vi "Ext.vi"(8 "error in (no error)":errorcluster, 9 "Val":variant, 10 "Tag":u16, 11 "Pulse in":refnum<class "Rigol DG822 Pulse.lvclass">) -> (0 "error out":errorcluster, 1 "Parsed":variant, 3 "Pulse out":refnum<class "Rigol DG822 Pulse.lvclass">)   [LabVIEW 2021, in "Rigol DG822 UI.lvlib" / "Rigol DG822 Pulse.lvlib" / "Rigol DG822 Pulse.lvclass"]
uses:
  Rigol DG822 Pulse.lvclass
  Rigol DG822 UI/lib/controls.llb/WaveformExtCall.ctl
  Rigol DG822 UI/lib/controls.llb/WaveformParamTags.ctl
  Rigol DG822 Pulse.lvclass/Rigol DG822 Pulse.ctl
  Rigol DG822 UI/lib/controls.llb/AllWaveformDataCluster.ctl
  Rigol DG822 UI/lib/controls.llb/DataCluster.ctl
  Rigol DG822 UI/lib/controls.llb/FT Controls Cluster.ctl
  Rigol DG822 UI/lib/controls.llb/String Indicators Cluster.ctl
  General/Files/lvlibp/Actors.lvlibp/Actors/Actors/Actors.lvclass
  D:/LabVIEW/General/Files/lvlibp/Actors.lvlibp/Actors/Actors/Actors.lvclass
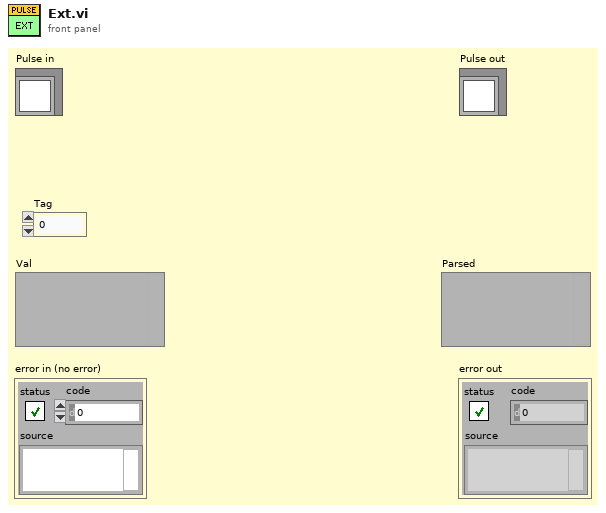
[diagram p1: front panel]
types:
  T1 = typedef "WaveformExtCall.ctl" = enum16{"Freq", "Period", "Ampl", "HighL", "Offset", "LowL", "Phase", "Duty", "Width", "RisEdge", "FallEdge", "Home", "InitData"}
  T2 = typedef "WaveformParamTags.ctl" = enum16{"Freq", "Period", "Ampl", "HighL", "Offset", "LowL", "Phase", "Duty", "Width", "RisEdge", "FallEdge"}
  T3 = cluster{"ParamTags":T2, "ParamTags 2":T2, "ParamTags 3":T2}
  T4 = typedef "AllWaveformDataCluster.ctl" = cluster{"Data":T5, "F/T Ctrls":T6, "String Indcs":T7}
  T5 = typedef "DataCluster.ctl" = cluster{"Freq":cluster{"Freq":dbl, "FreqUnit":enum32{"No Selection", "MHz", "kHz", "Hz", "mHz", "uHz"}, "FreqUnitPrcs":dbl}, "Period":cluster{"Period":dbl, "PeriodUnit":enum32{"No Selection", "s", "ms", "us", "ns"}, "PeriodUnitPrcs":dbl}, "Ampl":cluster{"Ampl":dbl, "AmplUnit":enum32{"No Selection", "Vpp", "mVpp"}, "AmplUnitPrcs":dbl}, "HighL":cluster{"HighL":dbl, "HighLUnit":enum32{"No Selection", "V", "mV"}, "HighLUnitPrcs":dbl}, "Offset":cluster{"Offset":dbl, "OffsetUnit":enum32{"No Selection", "Vdc", "mVdc"}, "OffsetUnitPrcs":dbl}, "LowL":cluster{"LowL":dbl, "LowLUnit":enum32{"No Selection", "V", "mV"}, "LowLUnitPrcs":dbl}, "Phase":cluster{"Phase":dbl, "PhaseUnit":enum32{"°"}, "PhaseUnitPrcs":dbl}, "Duty":cluster{"Duty":dbl, "DutyUnit":enum32{"%"}, "DutyUnitPrcs":dbl}, "Width":cluster{"Width":dbl, "WidthUnit":enum32{"No Selection", "s", "ms", "us", "ns"}, "WidthUnitPrcs":dbl}, "RisEdge":cluster{"RisEdge":dbl, "RisEdgeUnit":enum32{"No Selection", "s", "ms", "us", "ns"}, "RisEdgeUnitPrcs":dbl}, "FallEdge":cluster{"FallEdge":dbl, "FallEdgeUnit":enum32{"No Selection", "s", "ms", "us", "ns"}, "FallEdgeUnitPrcs":dbl}}
  T6 = typedef "FT Controls Cluster.ctl" = cluster{"Freq/Period":bool, "Ampl/HighL":bool, "Offset/LowL":bool, "Duty/Width":bool}
  T7 = typedef "String Indicators Cluster.ctl" = cluster{"Freq-Period":string, "Ampl-HighL":string, "Offset-LowL":string, "Phase":string, "Duty-Width":string, "RisEdge":string, "FallEdge":string}
  T8 = cluster{"Width":dbl, "WidthUnit":enum32{"No Selection", "s", "ms", "us", "ns"}, "WidthUnitPrcs":dbl}
  T9 = cluster{"RisEdge":dbl, "RisEdgeUnit":enum32{"No Selection", "s", "ms", "us", "ns"}, "RisEdgeUnitPrcs":dbl}
  T10 = cluster{"FallEdge":dbl, "FallEdgeUnit":enum32{"No Selection", "s", "ms", "us", "ns"}, "FallEdgeUnitPrcs":dbl}
  T11 = cluster{"Freq":dbl, "FreqUnit":enum32{"No Selection", "MHz", "kHz", "Hz", "mHz", "uHz"}, "FreqUnitPrcs":dbl}
  T12 = cluster{"Period":dbl, "PeriodUnit":enum32{"No Selection", "s", "ms", "us", "ns"}, "PeriodUnitPrcs":dbl}
  T13 = cluster{"Duty":dbl, "DutyUnit":enum32{"%"}, "DutyUnitPrcs":dbl}
  T14 = cluster{"Freq":cluster{"Freq":dbl, "FreqUnit":enum32{"No Selection", "MHz", "kHz", "Hz", "mHz", "uHz"}, "FreqUnitPrcs":dbl}, "Period":cluster{"Period":dbl, "PeriodUnit":enum32{"No Selection", "s", "ms", "us", "ns"}, "PeriodUnitPrcs":dbl}, "Duty":cluster{"Duty":dbl, "DutyUnit":enum32{"%"}, "DutyUnitPrcs":dbl}, "Width":cluster{"Width":dbl, "WidthUnit":enum32{"No Selection", "s", "ms", "us", "ns"}, "WidthUnitPrcs":dbl}, "RisEdge":cluster{"RisEdge":dbl, "RisEdgeUnit":enum32{"No Selection", "s", "ms", "us", "ns"}, "RisEdgeUnitPrcs":dbl}, "FallEdge":cluster{"FallEdge":dbl, "FallEdgeUnit":enum32{"No Selection", "s", "ms", "us", "ns"}, "FallEdgeUnitPrcs":dbl}}
  T15 = cluster{"Ampl":dbl, "AmplUnit":enum32{"No Selection", "Vpp", "mVpp"}, "AmplUnitPrcs":dbl}
  T16 = cluster{"HighL":dbl, "HighLUnit":enum32{"No Selection", "V", "mV"}, "HighLUnitPrcs":dbl}
  T17 = cluster{"Offset":dbl, "OffsetUnit":enum32{"No Selection", "Vdc", "mVdc"}, "OffsetUnitPrcs":dbl}
  T18 = cluster{"LowL":dbl, "LowLUnit":enum32{"No Selection", "V", "mV"}, "LowLUnitPrcs":dbl}
  T19 = cluster{"Ampl":cluster{"Ampl":dbl, "AmplUnit":enum32{"No Selection", "Vpp", "mVpp"}, "AmplUnitPrcs":dbl}, "HighL":cluster{"HighL":dbl, "HighLUnit":enum32{"No Selection", "V", "mV"}, "HighLUnitPrcs":dbl}, "Offset":cluster{"Offset":dbl, "OffsetUnit":enum32{"No Selection", "Vdc", "mVdc"}, "OffsetUnitPrcs":dbl}, "LowL":cluster{"LowL":dbl, "LowLUnit":enum32{"No Selection", "V", "mV"}, "LowLUnitPrcs":dbl}}
  T20 = cluster{"Phase":dbl, "PhaseUnit":enum32{"°"}, "PhaseUnitPrcs":dbl}
  T21 = cluster{"Duty":cluster{"Duty":dbl, "DutyUnit":enum32{"%"}, "DutyUnitPrcs":dbl}, "Width":cluster{"Width":dbl, "WidthUnit":enum32{"No Selection", "s", "ms", "us", "ns"}, "WidthUnitPrcs":dbl}, "RisEdge":cluster{"RisEdge":dbl, "RisEdgeUnit":enum32{"No Selection", "s", "ms", "us", "ns"}, "RisEdgeUnitPrcs":dbl}, "FallEdge":cluster{"FallEdge":dbl, "FallEdgeUnit":enum32{"No Selection", "s", "ms", "us", "ns"}, "FallEdgeUnitPrcs":dbl}}
  T22 = cluster{"RisEdge":cluster{"RisEdge":dbl, "RisEdgeUnit":enum32{"No Selection", "s", "ms", "us", "ns"}, "RisEdgeUnitPrcs":dbl}, "FallEdge":cluster{"FallEdge":dbl, "FallEdgeUnit":enum32{"No Selection", "s", "ms", "us", "ns"}, "FallEdgeUnitPrcs":dbl}}
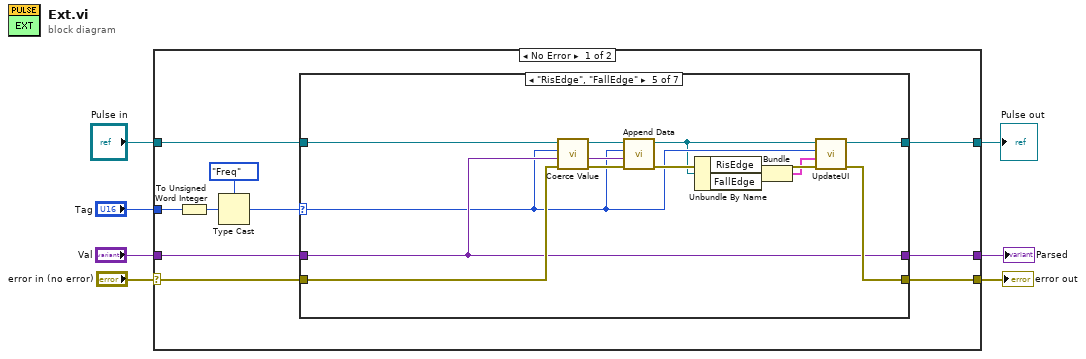
[diagram p0: block diagram]
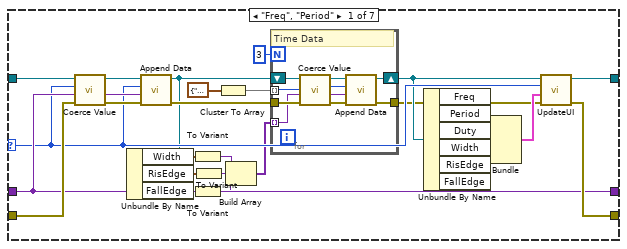
[diagram p2: hidden frame]
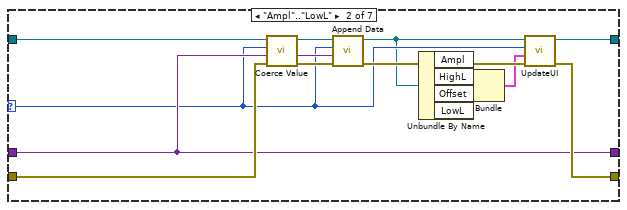
[diagram p3: hidden frame]
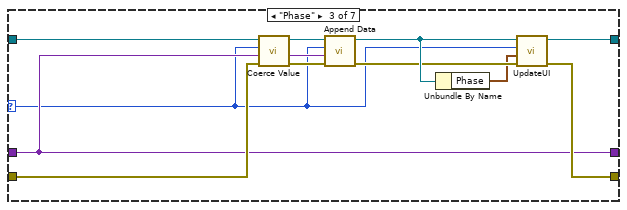
[diagram p4: hidden frame]
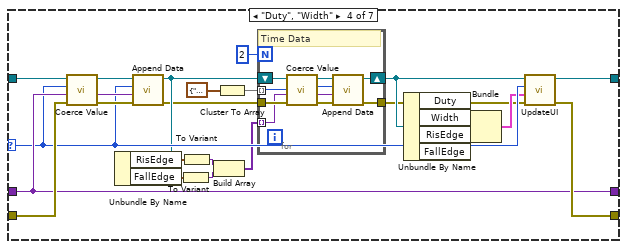
[diagram p5: hidden frame]
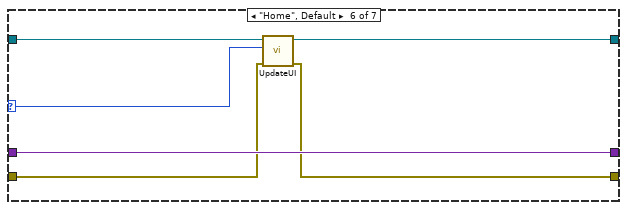
[diagram p6: hidden frame]
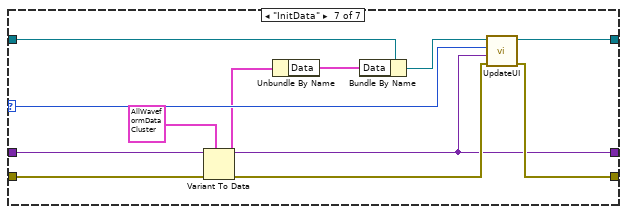
[diagram p7: hidden frame]
diagram:
  n1 = case shown="No Error" "error in (no error)" {
    selector: "error in (no error)" -> [w10 w152]
    tunnel: [w12 w151] -> w3
    tunnel: "Pulse in" -> [w13 w151]
    tunnel: "Tag" -> [w16 _]
    tunnel: "Val" -> [w15 _]
    tunnel: [w11 _] -> w2
    tunnel: [w9 w152] -> w1
    frame No Error {
      n2 = To Unsigned Word Integer(number=w16) -> (unsigned 16bit integer=w17:u16)
      n3 = Type Cast(type=WaveformExtCall."Freq" ("Enum"), x=w17) -> (*(type *) &x=w14:T1)
      n4 = case shown="\"RisEdge\", \"FallEdge\"" w14 {
        selector: w14 -> [w40 w63 w74 w102 w124 w137 w149]
        tunnel: w15 -> [w43 w67 w78 w105 w128 w136 w143]
        tunnel: w13 -> [w45 w69 w80 w107 w130 w139 w147]
        tunnel: [w47 w72 w84 w110 w133 w138 w150] -> w12
        tunnel: [w43 w67 w78 w105 w128 w136 w143] -> w11
        tunnel: w10 -> [w44 w68 w79 w106 w129 w135 w145]
        tunnel: [w46 w71 w83 w109 w132 w134 w148] -> w9
        frame "Freq", "Period" {
          n5 = call-dynamic "Coerce Value.vi"("error in (no error)"=w44, "Value"=w43, "ParamTags"=w40, "Rigol DG822 Pulse in"=w45) -> ("error out"=w41:errorcluster, "Coerced Value"=w42:variant, "Rigol DG822 Pulse out"=w22:refnum<class "Rigol DG822 Pulse.lvclass">)  [unwired: 5 in]
          n6 = call-dynamic "Append Data.vi"("error in (no error)"=w41, "Data"=w42, "ParamTags"=w40, "Rigol DG822 Pulse in"=w22) -> ("error out"=w29:errorcluster, "Rigol DG822 Pulse out"=w21:refnum<class "Rigol DG822 Pulse.lvclass">)  [unwired: 6 in]
          n7 = Unbundle By Name(w21) -> ("Width"=w23:T8, "RisEdge"=w25:T9, "FallEdge"=w24:T10)
          n8 = To Variant(anything=w23) -> (Variant=w19:variant)
          n9 = To Variant(anything=w24) -> (Variant=w18:variant)
          n10 = To Variant(anything=w25) -> (Variant=w20:variant)
          n11 = Cluster To Array(cluster=T3 {"ParamTags"=enum."Width", "ParamTags 2"=enum."RisEdge", "ParamTags 3"=enum."FallEdge"}) -> (array=w27:T2[])
          n12 = Build Array(w19, w20, w18) -> (w26:variant[])
          n13 = for {
            N: 3 -> [_]
            tunnel: [w51] -> w30
            shift-right: [w52] -> w31
            shift-left: w21 -> [w53]
            tunnel: w29 -> [w50]
            tunnel: w27 -> [w49] mode=indexing
            tunnel: w26 -> [w48] mode=indexing
            # "Time Data"
            n14 = call-dynamic "Coerce Value.vi"("error in (no error)"=w50, "Value"=w48, "ParamTags"=w49, "Rigol DG822 Pulse in"=w53) -> ("error out"=w54:errorcluster, "Coerced Value"=w55:variant, "Rigol DG822 Pulse out"=w56:refnum<class "Rigol DG822 Pulse.lvclass">)  [unwired: 5 in]
            n15 = call-dynamic "Append Data.vi"("error in (no error)"=w54, "Data"=w55, "ParamTags"=w49, "Rigol DG822 Pulse in"=w56) -> ("error out"=w51:errorcluster, "Rigol DG822 Pulse out"=w52:refnum<class "Rigol DG822 Pulse.lvclass">)  [unwired: 6 in]
          }
          n16 = Unbundle By Name(w31) -> ("Freq"=w38:T11, "Period"=w37:T12, "Duty"=w33:T13, "Width"=w36:T8, "RisEdge"=w35:T9, "FallEdge"=w34:T10)
          n17 = Bundle("Freq"=w38, "Period"=w37, "Duty"=w33, "Width"=w36, "RisEdge"=w35, "FallEdge"=w34) -> (w39:T14)  [unwired: 1 in]
          n18 = call "UpdateUI.vi"("error in (no error)"=w30, "Data"=w39, "Type"=w40, "Recursive in"=w31) -> ("error out"=w46:errorcluster, "Recursive out"=w47:refnum<class "Rigol DG822 Pulse.lvclass">)  [unwired: 6 in]
        }
        frame "Ampl".."LowL" {
          n19 = call-dynamic "Coerce Value.vi"("error in (no error)"=w68, "Value"=w67, "ParamTags"=w63, "Rigol DG822 Pulse in"=w69) -> ("error out"=w65:errorcluster, "Coerced Value"=w66:variant, "Rigol DG822 Pulse out"=w70:refnum<class "Rigol DG822 Pulse.lvclass">)  [unwired: 5 in]
          n20 = call-dynamic "Append Data.vi"("error in (no error)"=w65, "Data"=w66, "ParamTags"=w63, "Rigol DG822 Pulse in"=w70) -> ("error out"=w64:errorcluster, "Rigol DG822 Pulse out"=w57:refnum<class "Rigol DG822 Pulse.lvclass">)  [unwired: 6 in]
          n21 = Unbundle By Name(w57) -> ("Ampl"=w62:T15, "HighL"=w59:T16, "Offset"=w58:T17, "LowL"=w60:T18)
          n22 = Bundle("Ampl"=w62, "HighL"=w59, "Offset"=w58, "LowL"=w60) -> (w61:T19)  [unwired: 1 in]
          n23 = call "UpdateUI.vi"("error in (no error)"=w64, "Data"=w61, "Type"=w63, "Recursive in"=w57) -> ("error out"=w71:errorcluster, "Recursive out"=w72:refnum<class "Rigol DG822 Pulse.lvclass">)  [unwired: 6 in]
        }
        frame "Phase" {
          n24 = call-dynamic "Coerce Value.vi"("error in (no error)"=w79, "Value"=w78, "ParamTags"=w74, "Rigol DG822 Pulse in"=w80) -> ("error out"=w76:errorcluster, "Coerced Value"=w77:variant, "Rigol DG822 Pulse out"=w81:refnum<class "Rigol DG822 Pulse.lvclass">)  [unwired: 5 in]
          n25 = call-dynamic "Append Data.vi"("error in (no error)"=w76, "Data"=w77, "ParamTags"=w74, "Rigol DG822 Pulse in"=w81) -> ("error out"=w75:errorcluster, "Rigol DG822 Pulse out"=w82:refnum<class "Rigol DG822 Pulse.lvclass">)  [unwired: 6 in]
          n26 = Unbundle By Name(w82) -> ("Phase"=w73:T20)
          n27 = call "UpdateUI.vi"("error in (no error)"=w75, "Data"=w73, "Type"=w74, "Recursive in"=w82) -> ("error out"=w83:errorcluster, "Recursive out"=w84:refnum<class "Rigol DG822 Pulse.lvclass">)  [unwired: 6 in]
        }
        frame "Duty", "Width" {
          n28 = call-dynamic "Coerce Value.vi"("error in (no error)"=w106, "Value"=w105, "ParamTags"=w102, "Rigol DG822 Pulse in"=w107) -> ("error out"=w103:errorcluster, "Coerced Value"=w104:variant, "Rigol DG822 Pulse out"=w108:refnum<class "Rigol DG822 Pulse.lvclass">)  [unwired: 5 in]
          n29 = call-dynamic "Append Data.vi"("error in (no error)"=w103, "Data"=w104, "ParamTags"=w102, "Rigol DG822 Pulse in"=w108) -> ("error out"=w86:errorcluster, "Rigol DG822 Pulse out"=w87:refnum<class "Rigol DG822 Pulse.lvclass">)  [unwired: 6 in]
          n30 = Unbundle By Name(w87) -> ("RisEdge"=w92:T9, "FallEdge"=w91:T10)
          n31 = To Variant(anything=w91) -> (Variant=w89:variant)
          n32 = To Variant(anything=w92) -> (Variant=w90:variant)
          n33 = Build Array(w90, w89) -> (w88:variant[])
          n34 = Cluster To Array(cluster=cluster{"ParamTags 2":T2, "ParamTags 3":T2} {"ParamTags 2"=enum."RisEdge", "ParamTags 3"=enum."FallEdge"}) -> (array=w93:T2[])
          n35 = for {
            N: 2 -> [_]
            tunnel: [w114] -> w85
            shift-right: [w115] -> w95
            shift-left: w87 -> [w116]
            tunnel: w86 -> [w113]
            tunnel: w93 -> [w112] mode=indexing
            tunnel: w88 -> [w111] mode=indexing
            # "Time Data"
            n36 = call-dynamic "Coerce Value.vi"("error in (no error)"=w113, "Value"=w111, "ParamTags"=w112, "Rigol DG822 Pulse in"=w116) -> ("error out"=w117:errorcluster, "Coerced Value"=w118:variant, "Rigol DG822 Pulse out"=w119:refnum<class "Rigol DG822 Pulse.lvclass">)  [unwired: 5 in]
            n37 = call-dynamic "Append Data.vi"("error in (no error)"=w117, "Data"=w118, "ParamTags"=w112, "Rigol DG822 Pulse in"=w119) -> ("error out"=w114:errorcluster, "Rigol DG822 Pulse out"=w115:refnum<class "Rigol DG822 Pulse.lvclass">)  [unwired: 6 in]
          }
          n38 = Unbundle By Name(w95) -> ("Duty"=w101:T13, "Width"=w100:T8, "RisEdge"=w97:T9, "FallEdge"=w98:T10)
          n39 = Bundle("Duty"=w101, "Width"=w100, "RisEdge"=w97, "FallEdge"=w98) -> (w99:T21)  [unwired: 1 in]
          n40 = call "UpdateUI.vi"("error in (no error)"=w85, "Data"=w99, "Type"=w102, "Recursive in"=w95) -> ("error out"=w109:errorcluster, "Recursive out"=w110:refnum<class "Rigol DG822 Pulse.lvclass">)  [unwired: 6 in]
        }
        frame "RisEdge", "FallEdge" {
          n41 = call-dynamic "Coerce Value.vi"("error in (no error)"=w129, "Value"=w128, "ParamTags"=w124, "Rigol DG822 Pulse in"=w130) -> ("error out"=w126:errorcluster, "Coerced Value"=w127:variant, "Rigol DG822 Pulse out"=w131:refnum<class "Rigol DG822 Pulse.lvclass">)  [unwired: 5 in]
          n42 = call-dynamic "Append Data.vi"("error in (no error)"=w126, "Data"=w127, "ParamTags"=w124, "Rigol DG822 Pulse in"=w131) -> ("error out"=w125:errorcluster, "Rigol DG822 Pulse out"=w120:refnum<class "Rigol DG822 Pulse.lvclass">)  [unwired: 6 in]
          n43 = Unbundle By Name(w120) -> ("RisEdge"=w123:T9, "FallEdge"=w122:T10)
          n44 = Bundle("RisEdge"=w123, "FallEdge"=w122) -> (w121:T22)  [unwired: 1 in]
          n45 = call "UpdateUI.vi"("error in (no error)"=w125, "Data"=w121, "Type"=w124, "Recursive in"=w120) -> ("error out"=w132:errorcluster, "Recursive out"=w133:refnum<class "Rigol DG822 Pulse.lvclass">)  [unwired: 6 in]
        }
        frame "Home", Default {
          n46 = call "UpdateUI.vi"("error in (no error)"=w135, "Type"=w137, "Recursive in"=w139) -> ("error out"=w134:errorcluster, "Recursive out"=w138:refnum<class "Rigol DG822 Pulse.lvclass">)  [unwired: 7 in]
        }
        frame "InitData" {
          n47 = Variant To Data(error in=w145, type=T4 {"Data"={"Freq"={"Freq"=1.0, "FreqUnit"=enum."kHz", "FreqUnitPrcs"=9.0}, "Period"={"Period"=1.0, "PeriodUnit"=enum."ms", "PeriodUnitPrcs"=7.0}, "Ampl"={"Ampl"=5.0, "AmplUnit"=enum."Vpp", "AmplUnitPrcs"=4.0}, "HighL"={"HighL"=2.5, "HighLUnit"=enum."V", "HighLUnitPrcs"=4.0}, "Offset"={"Offset"=0.0, "OffsetUnit"=enum."Vdc", "OffsetUnitPrcs"=4.0}, "LowL"={"LowL"=-2.5, "LowLUnit"=enum."V", "LowLUnitPrcs"=4.0}, "Phase"={"Phase"=0.0, "PhaseUnit"=enum."°", "PhaseUnitPrcs"=3.0}, "Duty"={"Duty"=50.0, "DutyUnit"=enum."%", "DutyUnitPrcs"=3.0}, "Width"={"Width"=500.0, "WidthUnit"=enum."us", "WidthUnitPrcs"=4.0}, "RisEdge"={"RisEdge"=10.0, "RisEdgeUnit"=enum."ns", "RisEdgeUnitPrcs"=1.0}, "FallEdge"={"FallEdge"=10.0, "FallEdgeUnit"=enum."ns", "FallEdgeUnitPrcs"=1.0}}, "F/T Ctrls"={"Freq/Period"=FALSE, "Ampl/HighL"=FALSE, "Offset/LowL"=FALSE, "Duty/Width"=FALSE}, "String Indcs"={"Freq-Period"="1.000,000,000 kHz", "Ampl-HighL"="5.000,0 Vpp", "Offset-LowL"="0.000,0 Vdc", "Phase"="0.000 °", "Duty-Width"="50.000 %", "RisEdge"="10.0 ns", "FallEdge"="10.0 ns"}} ("Params Data"), Variant=w143) -> (data=w141:T4, error out=w144:errorcluster)
          n48 = Unbundle By Name(w141) -> ("Data"=w142:T5)
          n49 = Bundle By Name(cluster=w147, "Data"=w142) -> (w146:refnum<class "Rigol DG822 Pulse.lvclass">)
          n50 = call "UpdateUI.vi"("error in (no error)"=w144, "Data"=w143, "Type"=w149, "Recursive in"=w146) -> ("error out"=w148:errorcluster, "Recursive out"=w150:refnum<class "Rigol DG822 Pulse.lvclass">)  [unwired: 6 in]
        }
      }
    }
    frame Error {
    }
  }
  "error out" <- w1
  "Pulse out" <- w3
  "Parsed" <- w2
